vi "DCV Sub Panel.vi"(8 "error in":T2, 11 "GPIB address":string="16") -> (0 "error out":T2)   [LabVIEW 2017]
panel:
  out "Numeric":dbl
  in  "range value (volts)":dbl=1000.0 min=0.2 max=1000.0 format="%^.2e"
  in  "range (auto:0)":u16(ring) items=["autorange", "autorange once", "set min range", "set max range", "set range value"]
  in  "dig. filter count":dbl=10.0 min=1.0 max=100.0 step=1.0 format="%^.2e"
  in  "digital filter (off:0)":u16(ring) items=["off", "auto filter", "auto filter once", "moving filter", "repeating filter"]
  in  "integration time (0:auto)":u16(ring) items=["automatic", "automatic once", "set to minimum", "set to maximum", "set aperature value", "set NPLC value"]
  in  "integ. value":dbl=0.01667 format="%^.2e"
  in  "advanced filter (off:0)":u16(ring) items=["off", "enabled"]
  in  "resolution (4.5 digits:3)":u16(ring)=3 items=["auto resolution", "auto resolution once", "3.5 digits", "4.5 digits", "5.5 digits", "6.5 digits", "7.5 digits", "8.5 digits"]
  in  "noise tolerance (%)":dbl=1.0 min=0.0 max=100.0 step=1.0 format="%^.2e"
  in  "reference (off:0)":u16(ring) items=["off", "set reference value"]
  in  "reference value (volts)":dbl min=-1100.0 max=1100.0 format="%^.2e"
  in  "Tab Control":T1(tab)
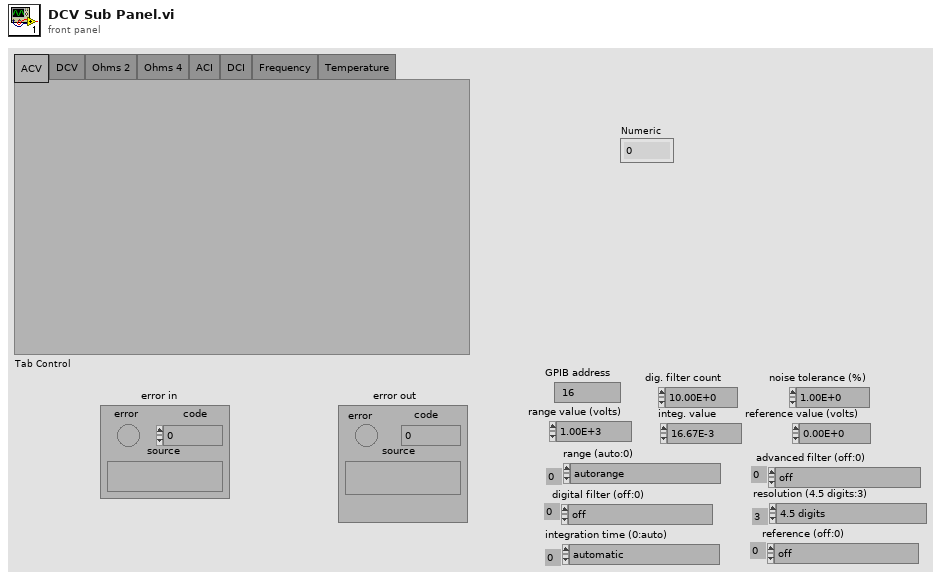
[diagram p1: front panel]
types:
  T1 = enum32{"ACV", "DCV", "Ohms 2", "Ohms 4", "ACI", "DCI", "Frequency", "Temperature"}
  T2 = cluster{"error":bool, "code":i32, "source":string}
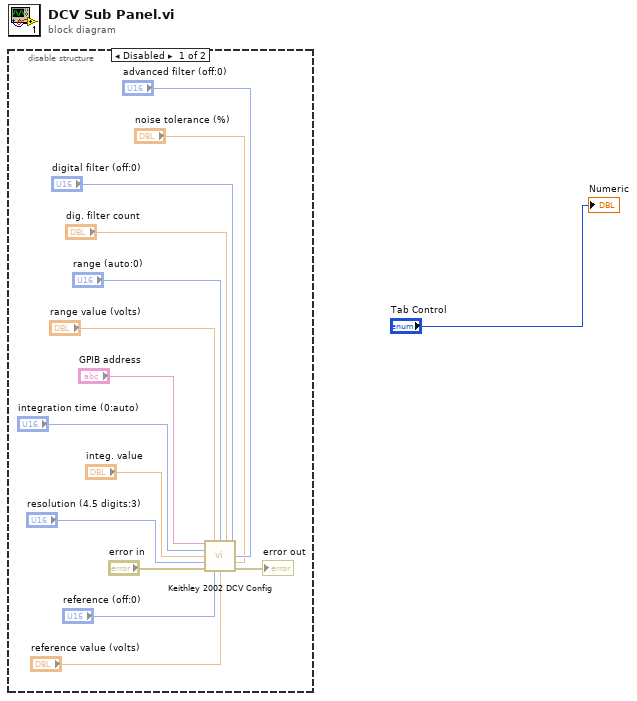
[diagram p0: block diagram]
diagram:
  n1 = disable-structure shown="Disabled" {
    frame Disabled {
      n2 = call "Keithley 2002 DCV Config.vi"("GPIB address"="GPIB address", "range value (volts)"="range value (volts)", "range (auto:0)"="range (auto:0)", "dig. filter count"="dig. filter count", "digital filter (off:0)"="digital filter (off:0)", "integration time (0:auto)"="integration time (0:auto)", "integ. value"="integ. value", "advanced filter (off:0)"="advanced filter (off:0)", "resolution (4.5 digits:3)"="resolution (4.5 digits:3)", "noise tolerance (%)"="noise tolerance (%)", "error in"="error in", "reference (off:0)"="reference (off:0)", "reference value (volts)"="reference value (volts)") -> ("error out"=→"error out":T2)  [unwired: 2 in]
    }
    frame Enabled {
    }
  }
  "Numeric" <- "Tab Control"
